vi "Calculate Distance XY.vi"(9 "Y":dbl, 11 "X":dbl) -> (3 "DIST Out":dbl)   [LabVIEW 2020, in "Swerve_Odometry_SEN.lvlib"]
doc: "Utility function to calculate distance (hypotenuse) result = ( x ^2 + y ^2 ) ^ 0.5\n\nParameters:\n - X\n - Y\n\nResult\n - Distance"
uses:
  Swerve_Odometry_SEN.lvlib
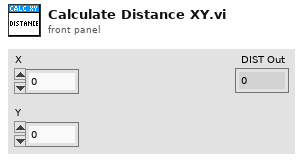
[diagram p1: front panel]
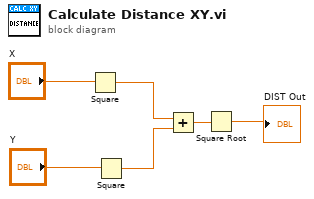
[diagram p0: block diagram]
diagram:
  n1 = Square(x="X") -> (x^2=w4:dbl)
  n2 = Square(x="Y") -> (x^2=w3:dbl)
  n3 = Add(x=w4, y=w3) -> (x+y=w2:dbl)
  n4 = Square Root(x=w2) -> (sqrt(x)=→"DIST Out":dbl)
